vi "Listbox_Init.vi"(3 "Container State":T5, 4 "Previous State":variant, 5 "Previous Version":T4) -> (2 "Current State":T1)   [LabVIEW 2012, in "ListBox_XControl.xctl"]
uses:
  ListBox_XControl.xctl
  ListBox_State.ctl
  VIs/Order Type Def.ctl
  VIs/Value Filters.ctl
  <vilib>/_xctls/Container State.ctl
  <vilib>/_xctls/Version.ctl
  <vilib>/_xctls/XControlSupport.lvlib
panel:
  in  "Default Indicator State":T1={"Alternating BG Color"=13359335, "Alternating Text Color"=0, "Order by Col"=0, "Order"=enum."Off", "Value Filters"=[], "Item Names before Filtering"=[], "Item Names after Filtering"=[], "Column Header Strings[]"=[], "Column Widths"=[], "Autosize by Column"=0, "Autosize Activated?"=FALSE, "Autosize Cell Padding"=0}
  in  "Default Control State":T1={"Alternating BG Color"=13359335, "Alternating Text Color"=0, "Order by Col"=0, "Order"=enum."Off", "Value Filters"=[], "Item Names before Filtering"=[], "Item Names after Filtering"=[], "Column Header Strings[]"=[], "Column Widths"=[], "Autosize by Column"=0, "Autosize Activated?"=FALSE, "Autosize Cell Padding"=0}
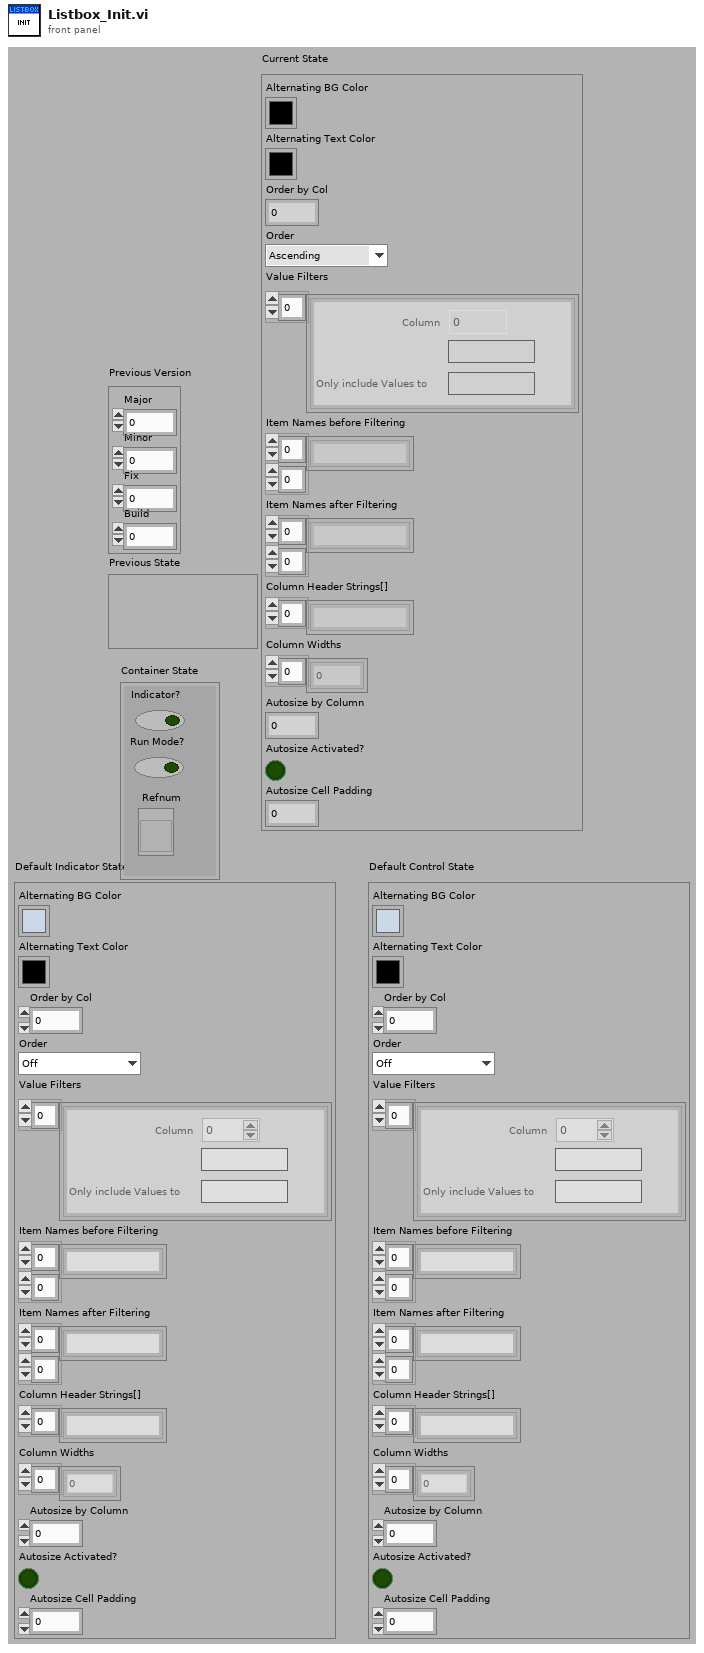
[diagram p1: front panel]
types:
  T1 = typedef "ListBox_XControl.xctl/ListBox_State.ctl" = cluster{"Alternating BG Color":u32, "Alternating Text Color":u32, "Order by Col":i32, "Order":T2, "Value Filters":T3, "Item Names before Filtering":string[][], "Item Names after Filtering":string[][], "Column Header Strings[]":string[], "Column Widths":u32[], "Autosize by Column":i32, "Autosize Activated?":bool, "Autosize Cell Padding":u32}
  T2 = typedef "ListBox_XControl.xctl/Order Type Def.ctl" = enum16{"Ascending", "Descending", "Off"}
  T3 = typedef "ListBox_XControl.xctl/Value Filters.ctl" = cluster{"Column":i32, "Only include Values From":string, "Only include Values to":string}[]
  T4 = typedef "XControlSupport.lvlib/Version.ctl" = cluster{"Major":u16, "Minor":u16, "Fix":u16, "Build":u16}
  T5 = typedef "XControlSupport.lvlib/Container State.ctl" = cluster{"Indicator?":bool, "Run Mode?":bool, " Refnum":refnum<vi>}
  T6 = typedef "ListBox_XControl.xctl/ListBox_State_1_1_0_0.ctl" = cluster{"Alternating BG Color":u32, "Alternating Text Color":u32, "Order by Col":i32, "Order":T2, "Value Filters":T3, "Item Names before Filtering":string[][], "Item Names after Filtering":string[][], "Column Header Strings[]":string[], "Column Widths":u32[]}
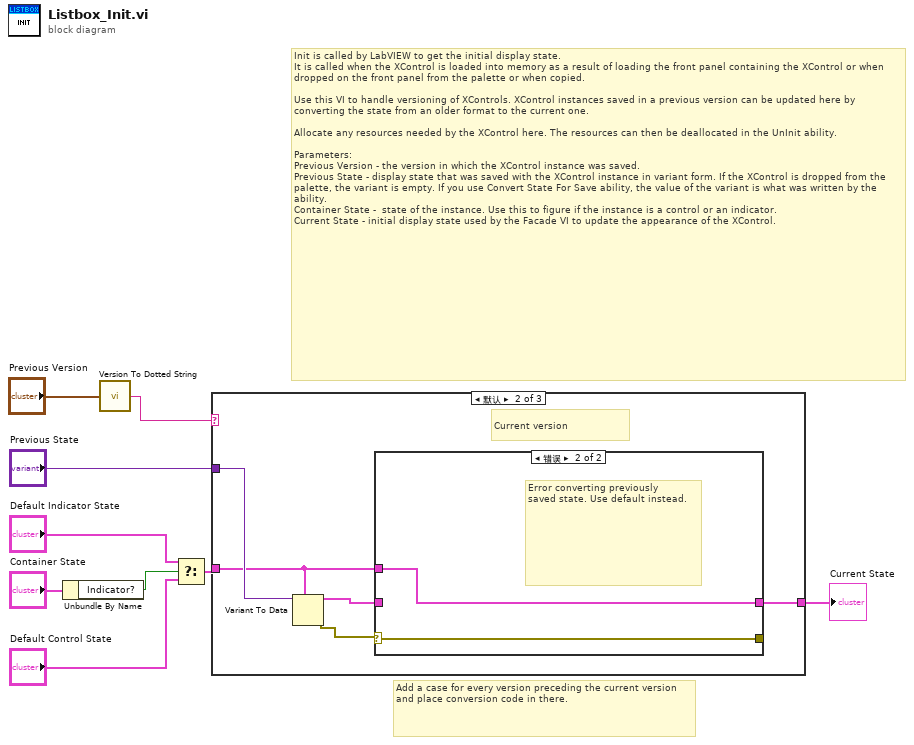
[diagram p0: block diagram]
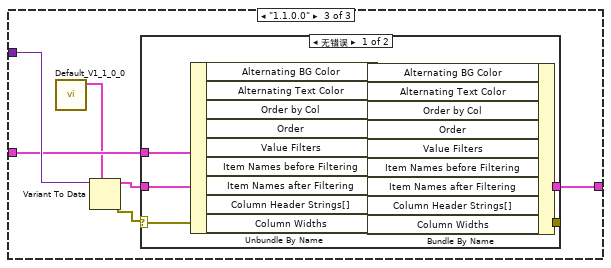
[diagram p4: hidden frame]
diagram:
  # "Add a case for every version preceding the current version and place conversion code in there."
  # "Init is called by LabVIEW to get the initial display state.\nIt is called when the XControl is loaded into memory as a result of loading the front panel containing the XControl or when dropped on the front panel from the palette or when copied.\n\nUse this VI to handle versioning of XControls. XControl instances saved in a previous version can be updated here by converting the state from an older format to the current one.\n\nAllocate any resources needed by the XControl here. The resources can then be deallocated in the UnInit ability.\n\nParameters:\nPrevious Version - the version in which the XControl instance was saved.\nPrevious State - display state that was saved with the XControl instance in variant form. If the XControl is dropped from the palette, the variant is empty. If you use Convert State For Save ability, the value of the variant is what was written by the ability. \nContainer State -  state of the instance. Use this to figure if the instance is a control or an indicator.\nCurrent State - initial display state used by the Facade VI to update the appearance of the XControl."
  n1 = Unbundle By Name("Container State") -> ("Indicator?"=w4:bool)
  n2 = call <vilib>:"Version To Dotted String.vi"("Version"="Previous Version") -> ("String Version"=w1:string)
  n3 = Select(t="Default Indicator State", s=w4, f="Default Control State") -> (s? t:f=w3:T1)
  n4 = case shown="默认" w1 {
    tunnel: "Previous State" -> [_ w15 w25]
    tunnel: [w10 w11 w21] -> w8
    tunnel: w3 -> [w10 w12 w22]
    frame "0.0.0.0" {
      # "Just created, use default state"
    }
    frame Default {
      # "Current version"
      n5 = Variant To Data(type=w12, Variant=w15) -> (data=w13:T1, error out=w14:errorcluster)  [unwired: 1 in]
      n6 = case shown="错误" w14 {
        selector: w14 -> [w17 w18]
        tunnel: w13 -> [w16 _]
        tunnel: [w16 w19] -> w11
        tunnel: w12 -> [_ w19]
        tunnel: [w17 w18] -> _
        frame No Error {
        }
        frame Error {
          # "Error converting previously \nsaved state. Use default instead."
        }
      }
    }
    frame "1.1.0.0" {
      n7 = call "Default_V1_1_0_0.vi"() -> ("State"=w20:T6)  [unwired: 11 in]
      n8 = Variant To Data(type=w20, Variant=w25) -> (data=w23:T6, error out=w24:errorcluster)  [unwired: 1 in]
      n9 = case shown="无错误" w24 {
        selector: w24 -> [w38 w39]
        tunnel: w23 -> [w36 _]
        tunnel: [w26 w40] -> w21
        tunnel: w22 -> [w37 w40]
        tunnel: [w38 w39] -> _
        frame No Error {
          n10 = Unbundle By Name(w36) -> ("Alternating BG Color"=w35:u32, "Alternating Text Color"=w34:u32, "Order by Col"=w33:i32, "Order"=w32:T2, "Value Filters"=w31:T3, "Item Names before Filtering"=w30:string[][], "Item Names after Filtering"=w29:string[][], "Column Header Strings[]"=w28:string[], "Column Widths"=w27:u32[])
          n11 = Bundle By Name(cluster=w37, "Alternating BG Color"=w35, "Alternating Text Color"=w34, "Order by Col"=w33, "Order"=w32, "Value Filters"=w31, "Item Names before Filtering"=w30, "Item Names after Filtering"=w29, "Column Header Strings[]"=w28, "Column Widths"=w27) -> (w26:T1)
        }
        frame Error {
          # "Error converting previously \nsaved state. Use default instead."
        }
      }
    }
  }
  "Current State" <- w8
